vi "ErrorMsg_LinkData.vi"() -> ()   [LabVIEW 2019]
panel:
  in  "Error Reset":refnum<vi>
  in  "ErrorMsg_Path":path
  in  "ErrorMsg_Exit":refnum<vi>
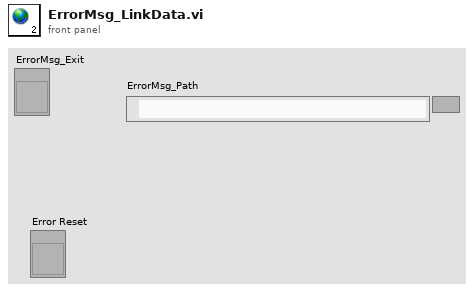
[diagram p1: front panel]
diagram:
